vi "PH_Cont-601k_PSU.set GUI Refs.vi"(0 "VI in":refnum<vi>, 1 "Class":string, 2 "GUI Refs":T1, 5 "error in (no error)":errorcluster) -> (14 "VI out":refnum<vi>, 19 "error out":errorcluster)   [LabVIEW 2014, in "PH_Cont-601k_PSU.lvlib"]
uses:
  PH_Cont-601k_PSU.lvlib
  PH_Cont-601k_PSU.GUI Refs.ctl
  PH_Cont-601k_PSU.Device Status.ctl
  PH_Cont-601k_PSU.Readyness.ctl
  PH_Cont-601k_PSU.Readyness Program.ctl
  PH_Cont-601k_PSU.Readyness Device.ctl
  PH_Cont-601k_PSU.Mode.ctl
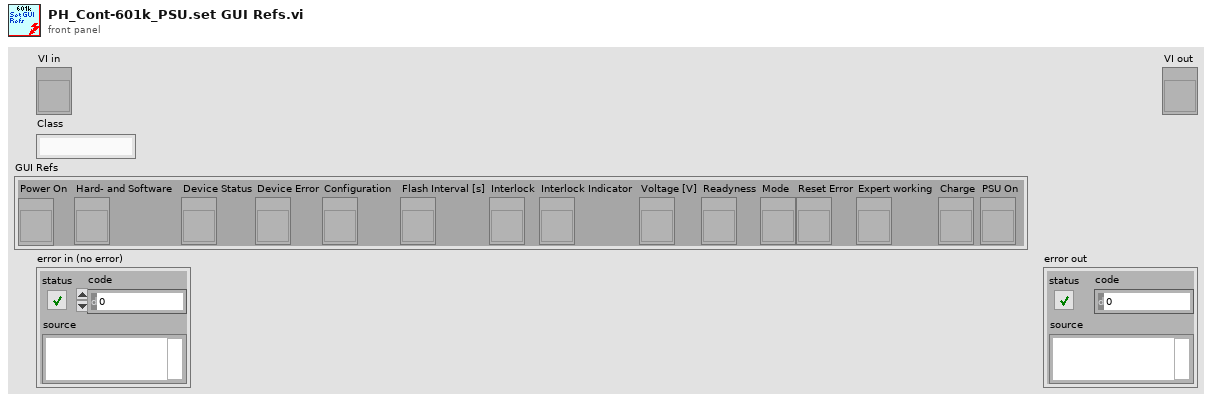
[diagram p1: front panel]
types:
  T1 = typedef "PH_Cont-601k_PSU.lvlib/PH_Cont-601k_PSU.GUI Refs.ctl" = cluster{"Power On":refnum<vi>, "Hard- and Software":refnum<vi>, "Device Status":refnum<vi>, "Device Error":refnum<vi>, "Configuration":refnum<vi>, "Flash Interval [s]":refnum<vi>, "Interlock":refnum<vi>, "Interlock Indicator":refnum<vi>, "Voltage [V]":refnum<vi>, "Readyness":refnum<vi>, "Mode":refnum<vi>, "Reset Error":refnum<vi>, "Expert working":refnum<vi>, "Charge":refnum<vi>, "PSU On":refnum<vi>}
  T2 = typedef "PH_Cont-601k_PSU.lvlib/PH_Cont-601k_PSU.i attribute.ctl" = cluster{"GUI Refs":T1, "Interlock":bool, "Service ID applied Voltage":i32, "Device Settings":cluster{"Configuration":T3, "Flash Interval [s]":dbl, "Mode":T4, "Voltage [V]":u16, "Charge":bool, "VISA resource name":refnum<visa-resource-name>}, "Readyness":T5, "Information":cluster{"VISA resource name":refnum<visa-resource-name>, "Tagname Power On":string, "Interlock":cluster{"Instance":string, "Tagname":string}, "Limits [V]":cluster{"Lower":dbl, "Upper":dbl}, "Tagname PSU On":string}, "R2S":bool, "Charge is allowed":bool}
  T3 = typedef "PH_Cont-601k_PSU.lvlib/PH_Cont-601k_PSU.Configuration.ctl" = u16
  T4 = typedef "PH_Cont-601k_PSU.lvlib/PH_Cont-601k_PSU.Mode.ctl" = enum32{"STOP", "STANDBY", "READY", "EMISSION", "ERROR"}
  T5 = typedef "PH_Cont-601k_PSU.lvlib/PH_Cont-601k_PSU.Readyness.ctl" = cluster{"Program":T6, "Device":T7}
  T6 = typedef "PH_Cont-601k_PSU.lvlib/PH_Cont-601k_PSU.Readyness Program.ctl" = enum32{"OFF", "POWER", "INTERLOCK"}
  T7 = typedef "PH_Cont-601k_PSU.lvlib/PH_Cont-601k_PSU.Readyness Device.ctl" = enum32{"OFF", "CONNECTING", "CONNECTED", "OPERATING", "EOC", "ERROR"}
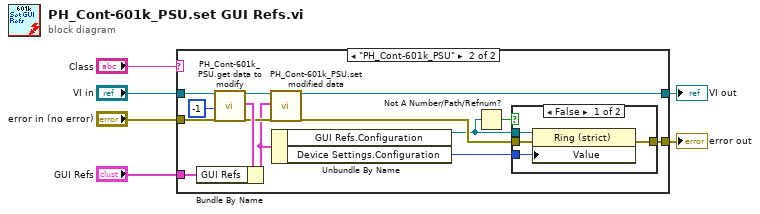
[diagram p0: block diagram]
diagram:
  n1 = case shown="\"PH_Cont-601k_PSU\"" "Class" {
    tunnel: [w7 w12] -> w6
    tunnel: [w8 w20] -> w5
    tunnel: "error in (no error)" -> [w7 w19]
    tunnel: "VI in" -> [w8 w18]
    tunnel: "GUI Refs" -> [_ w14]
    frame Default {
    }
    frame "PH_Cont-601k_PSU" {
      n2 = call "PH_Cont-601k_PSU.get data to modify.vi"("i ref in"=w18, "ms timeout (10000)"=-1, "error in (no error)"=w19) -> ("i ref out"=w15:refnum<vi>, "i attribute"=w22:T2, "error out"=w16:errorcluster)  [unwired: 13 in, 1 out]
      n3 = Bundle By Name(cluster=w22, "GUI Refs"=w14) -> (w13:T2)
      n4 = call "PH_Cont-601k_PSU.set modified data.vi"("i ref in"=w15, "i attribute"=w13, "error in (no error)"=w16) -> ("i ref out"=w20:refnum<vi>, "error out"=w21:errorcluster)  [unwired: 15 in]
      n5 = Unbundle By Name(w13) -> ("GUI Refs.Configuration"=w9:refnum<vi>, "Device Settings.Configuration"=w11:T3)
      n6 = Not A Number/Path/Refnum?(number/path/refnum=w9) -> (NaN/Path/Refnum?=w10:bool)
      n7 = case shown="False" w10 {
        tunnel: w21 -> [w26 w27]
        tunnel: [w25 w27] -> w12
        tunnel: w9 -> [w24 _]
        tunnel: w11 -> [w23 _]
        frame False {
          n8 = property class="Ring (strict)"(reference=w24, error in=w26, "Value"=w23) -> (error out=w25:errorcluster)  [unwired: 1 out]
        }
        frame True {
        }
      }
    }
  }
  "error out" <- w6
  "VI out" <- w5
